vi "BuildJPG.vi"(11 "image":string) -> (3 "new picture":picture)   [LabVIEW 2022 SP3]
panel:
  out "size(s)":i32
  out "slash codes ignored":u8[](array[numeric]) format="%.0x"
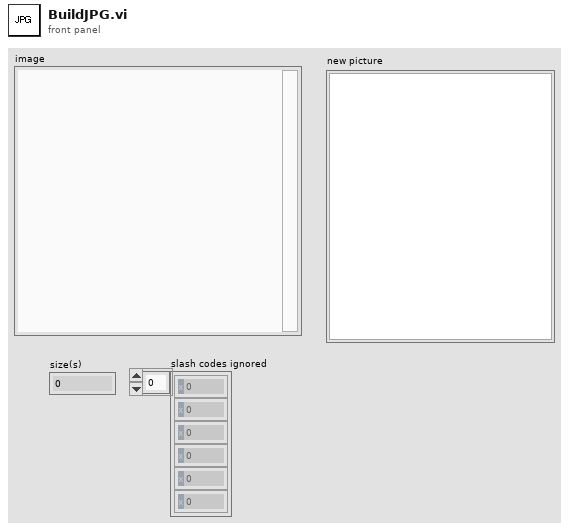
[diagram p1: front panel]
types:
  T1 = typedef "imagedata.ctl" = cluster{"image type":i32, "image depth":i32, "image":u8[], "mask":u8[], "colors":u32[], "Rectangle":cluster{"left":i16, "top":i16, "right":i16, "bottom":i16}}
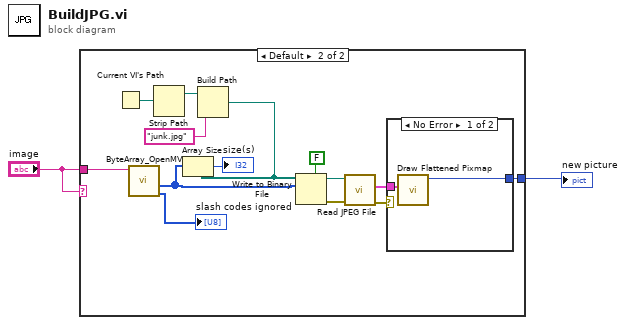
[diagram p0: block diagram]
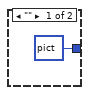
[diagram p2: hidden frame]
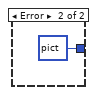
[diagram p3: hidden frame]
diagram:
  n1 = case shown="Default" "image" {
    tunnel: "image" -> [_ w7]
    tunnel: [picture data[5B] ("new picture") w5] -> w1
    frame "" {
    }
    frame Default {
      n2 = Current VI's Path() -> (path=w11:path)
      n3 = call "ByteArray_OpenMV.vi"("String"=w7) -> ("slash codes ignored"=→"slash codes ignored":u8[], "Array"=w12:u8[])  [unwired: 8 in, 1 out]
      n4 = Strip Path(path=w11) -> (stripped path=w9:path)  [unwired: 1 out]
      n5 = Array Size(array=w12) -> (size(s)=→"size(s)":i32)
      n6 = Build Path(base path=w9, name or relative path="junk.jpg" ("regular expression")) -> (appended path=w8:path)
      n7 = Write to Binary File(file (use dialog)=w8, data=w12, 5:FALSE ("prepend array or string size? (T)")) -> (error out=w13:errorcluster)  [unwired: 3 in, 2 out]
      n8 = call <vilib>:"Read JPEG File.vi"("error in (no error)"=w13, "path to JPEG file"=w8) -> ("error out"=w6:errorcluster, "image data"=w4:T1)  [unwired: 7 in, 1 out]
      n9 = case shown="No Error" w6 {
        tunnel: w4 -> [w18 _]
        tunnel: [w17 picture data[5B] ("new picture")] -> w5
        frame No Error {
          n10 = call <vilib>:"Draw Flattened Pixmap.vi"("image data"=w18) -> ("new picture"=w17:picture)  [unwired: 8 in]
        }
        frame Error {
        }
      }
    }
  }
  "new picture" <- w1
